vi "Universial XsYa.vi"() -> ()   [LabVIEW 2023]
uses:
  <vilib>/Utility/file.llb/Write Delimited Spreadsheet (DBL).vi
panel:
  in  "Status":enum32{"Measurement Status"}(tab)
  in  "Comments":string="See the below notes for this measurement.\n\nSR785 Status:Fre Span 51200.000000\n Hz; Center Fre 25600.000000\n Hz; Points(0 for 101, 1 for 201, 2 for 401 3 for 801): 2\n; Start, End Fre: 0.000000\n, 51200.000000\nHz; Unit y: dBVpk\n;\n"
  out "Current FIeld":dbl=0.5
  out "Current Current":dbl=2.5
  out "error out":errorcluster
  in  "Response Control":enum32{"cRIO slow V", "SR785"}(tab)=enum."SR785"
  in  "Channel":string(combo)="AI0"
  in  "Average":i32=1000
  out "FFT record time s":dbl=0.015625 caption="Delay Time (s)"
  in  "SR785 VISA":string="GPIB0::10::INSTR"
  in  "Display data":i32(ring) items=["Display A", "Display B"]
  in  "Center Hz":dbl=25000.0 format="%^.2e"
  in  "Span Hz":dbl=50000.0 format="%^.2e"
  in  "Resolution":i32(ring)=3 items=["100", "200", "400", "800"]
  out "CRIO pipe":T1={"DAQ_CMD_Writer endpoint"="DAQ_CMD_Writer", "DAQ_AI_Reader endpoint"="DAQ_AI_Reader", "vi reference"=refnum, "application reference"=refnum}
  in  "Excitation control":enum32{"B", "I"}(tab)
  in  "B Origin":dbl=-1.5 format="%#_13g"
  in  "B Radius":dbl=2.0 format="%#_13g"
  in  "B step":dbl=0.1 format="%#_13g"
  in  "B Ramp first":bool=TRUE
  in  "B Ramp type":string(combo)="Range"
  in  "Magnet Device Select":string(combo)="Elsa Magnet mT"
  in  "Field Rate mT per sec":dbl=0.1 format="%#_13g"
  in  "scale":dbl=1.0
  in  "I Origin":dbl format="%#_13g"
  in  "I step":dbl=0.05 format="%#_13g"
  in  "I Radius":dbl=2.5 format="%#_13g"
  in  "I Ramp first":bool=TRUE
  in  "I Ramp type":string(combo)="Range"
  in  "I Device Select":string(combo)="cRIO Slow"
  in  "AO Channel":string(combo)="AO0"
  in  "Book number":i32=684
  in  "parent data folder":path=path "C:/Users/gyue/Box/Guang Yue uiuc research box folder/data/Contour plot"
  # "This VI control measurements of multiple indenpent variable (Xs, such as B, I) and single channel data array (Yarray, FFT, V curve etc.)"
  # "Data structure: time-para.xml for all VI controls value, para.dat contains dimensions of data in form (x1 numbers, x2 numbers\\n y1 numbers, y2, numbers), field.dat contains lines of independent variables at each measurement, data.dat contains measurment data line, one measurement per line or group of lines."
  # "Attation: The actuall frequency may different from set value, check the Comments control."
  # "value in uA x scale=raw"
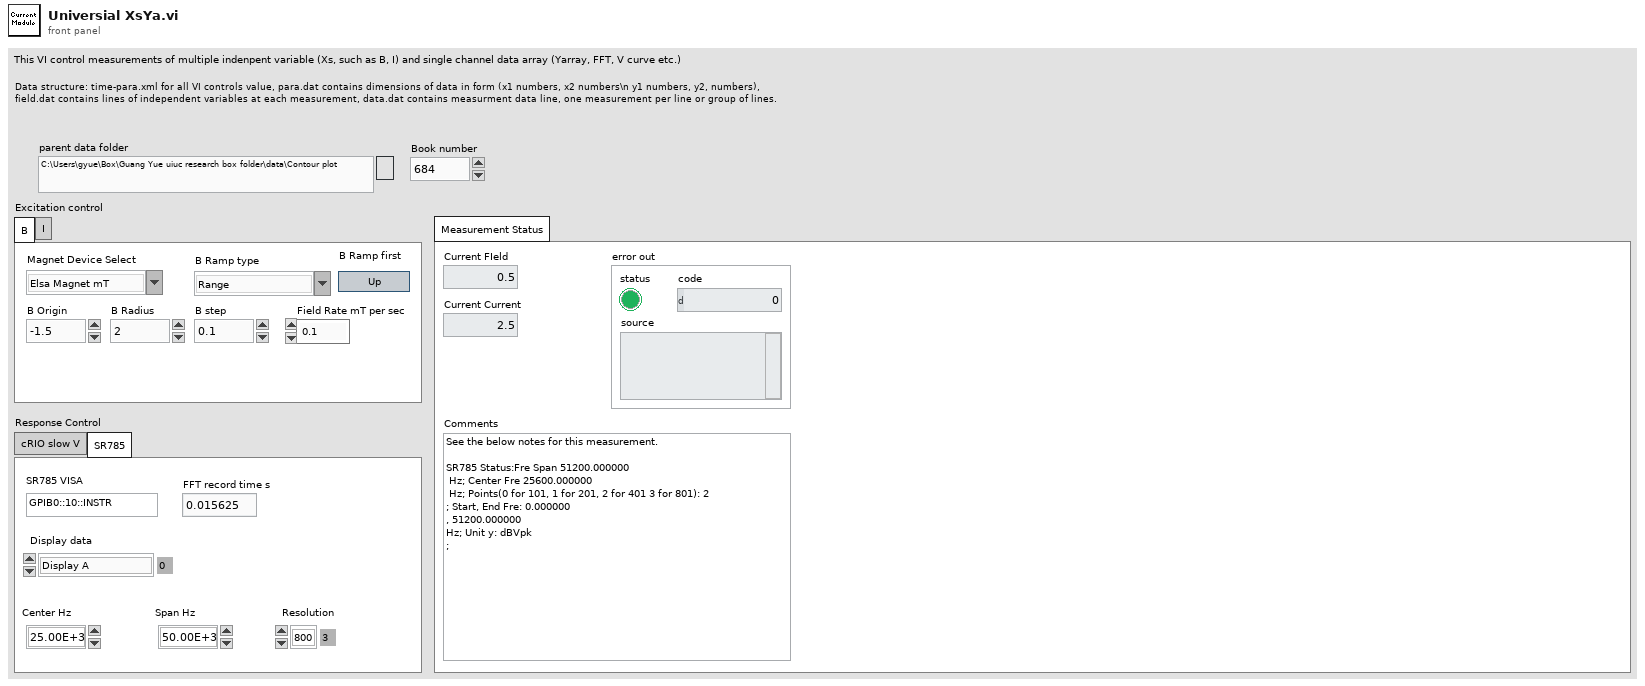
[diagram p1: front panel]
types:
  T1 = cluster{"DAQ_CMD_Writer endpoint":refnum<k21>, "DAQ_AI_Reader endpoint":refnum<k21>, "vi reference":refnum<vi>, "application reference":refnum<vi>}
  T2 = cluster{"AI0":dbl, "AI1":dbl, "AI2":dbl, "AI3":dbl}
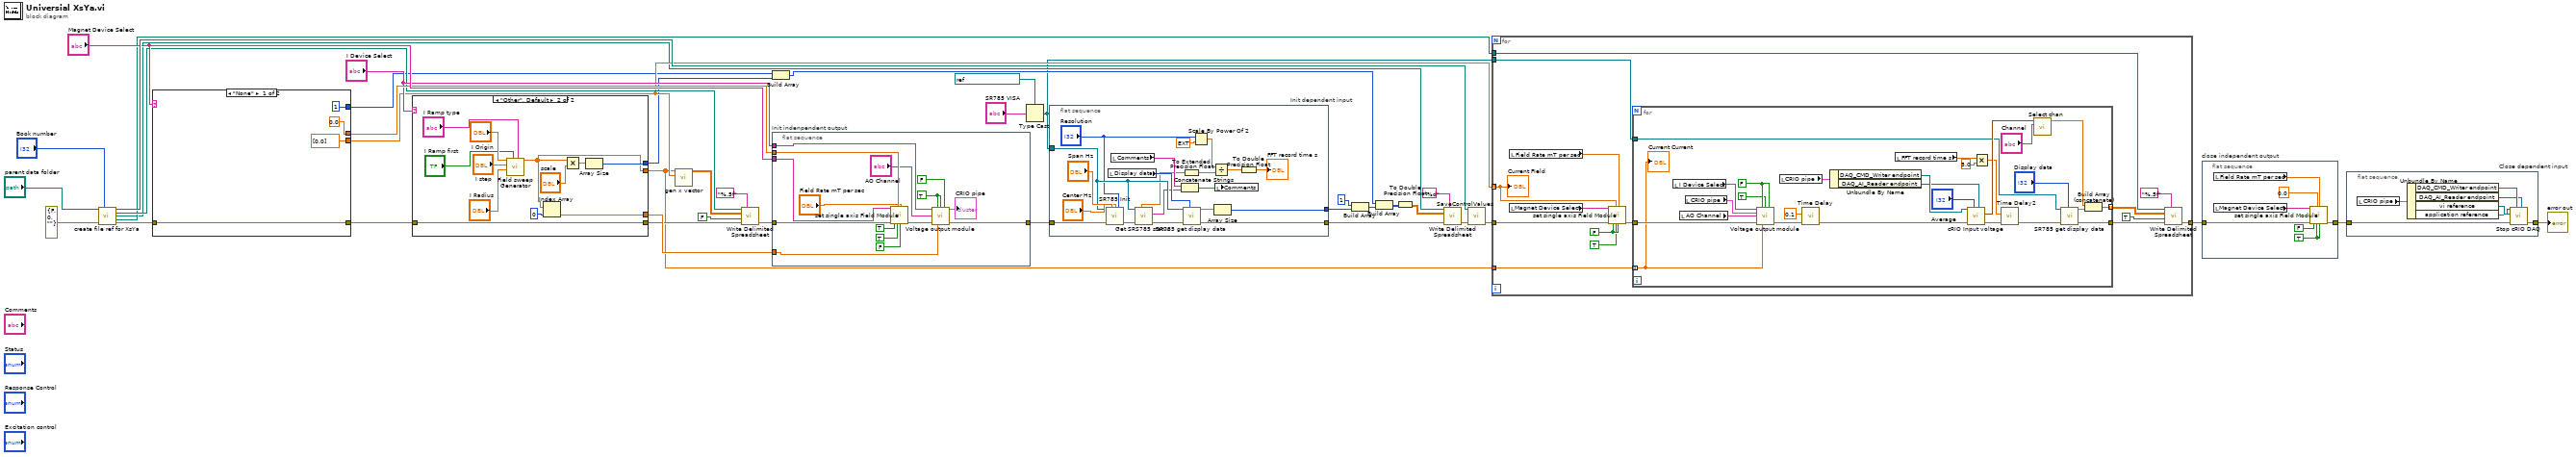
[diagram p0: block diagram]
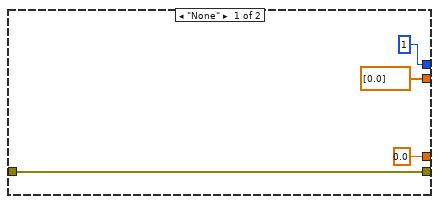
[diagram p2: hidden frame]
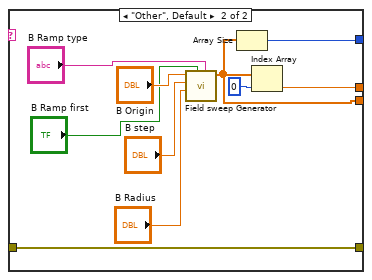
[diagram p3: hidden frame]
diagram:
  n1 = call "create file ref for XsYa.vi"("parent data folder"="parent data folder", "Book number"="Book number", "error in"=errorcluster {"status"=FALSE, "code"=0, "source"=""}) -> ("xml path"=w36:path, "field dat"=w27:path, "para dat"=w16:path, "data dat"=w21:path, "error out"=w3:errorcluster)  [unwired: 8 in]
  n2 = case shown="\"None\"" "Magnet Device Select" {
    tunnel: [0.0 w47] -> w34
    tunnel: w3 -> [w42 w46]
    tunnel: [w42 w46] -> w31
    tunnel: [dbl[] [0.0] ("output array") w45] -> w24
    tunnel: [1 w44] -> w14
    frame "None" {
    }
    frame "Other", Default {
      n3 = call "Field sweep Generator.vi"("Ramp type"="B Ramp type", "Ramp up first T"="B Ramp first", "Field Radius"="B Radius", "Field step"="B step", "Field Origin"="B Origin") -> ("output array"=w45:dbl[])  [unwired: 6 in]
      n4 = Array Size(array=w45) -> (size(s)=w44:i32)
      n5 = Index Array(array=w45, index=0) -> (element=w47:dbl)
    }
  }
  n6 = case shown="\"Other\", Default" "I Device Select" {
    tunnel: [0.0 w63] -> w32
    tunnel: w31 -> [w56 w62]
    tunnel: [w56 w62] -> w30
    tunnel: [dbl[] [0.0] ("output array") w58] -> w23
    tunnel: [1 w59] -> w13
    frame "None" {
    }
    frame "Other", Default {
      n7 = call "Field sweep Generator.vi"("Ramp type"="I Ramp type", "Ramp up first T"="I Ramp first", "Field Radius"="I Radius", "Field step"="I step", "Field Origin"="I Origin") -> ("output array"=w58:dbl[])  [unwired: 6 in]
      n8 = Index Array(array=w58, index=0) -> (element=w63:dbl)
      n9 = Multiply(x=w58, y="scale") -> (x*y=w60:dbl[])
      n10 = Array Size(array=w60) -> (size(s)=w59:i32)
    }
  }
  n11 = call "gen x vector.vi"("B"=w24, "I"=w23) -> ("Array"=w25:dbl[][])  [unwired: 9 in]
  n12 = call-poly <vilib>:"Write Delimited Spreadsheet.vi"("file path (dialog if empty)"=w27, "format (%.3f)"="%.5f", "2D data"=w25, "append to file? (new file:F)"=FALSE, "error in (no error)"=w30) -> ("error out"=w29:errorcluster)  [unwired: 9 in, 1 out]
  n13 = Build Array(w14, w13) -> (w12:i32[])
  n14 = flat-sequence "Init indenpendent output" {
    tunnel: w29 -> [w72]
    tunnel: w34 -> [w81]
    tunnel: "Magnet Device Select" -> [w80]
    tunnel: "I Device Select" -> [w79]
    tunnel: w32 -> [w78]
    tunnel: [w71] -> w22
    frame #0 {
      w77 = TRUE ("Init")
      n15 = call "set single axis Field Module.vi"("Field Device Select"=w80, "error in (no error)"=w72, "Init"=TRUE, "Field Target mT or dBm"=w81, "Exec"=TRUE, "Field Rate mT per sec"="Field Rate mT per sec", "final"=FALSE) -> ("error out"=w75:errorcluster)  [unwired: 12 in]
      n16 = call "Voltage output module.vi"("Device Select"=w79, "Init"=w77, "Exec"=w77, "finish up"=FALSE, "AO Channel"="AO Channel", "Error In"=w75, "Voltage"=w78) -> ("current Control pipe"=→"CRIO pipe":T1, "Error out"=w71:errorcluster)  [unwired: 7 in]
    }
  }
  n17 = Type Cast(type=refnum<visa-resource-name> "GPIB0::10::INSTR" ("SR785 VISA"), x="SR785 VISA") -> (*(type *) &x=w7:refnum<visa-resource-name>)
  n18 = flat-sequence "Init dependent input" {
    tunnel: w22 -> [w101]
    tunnel: [w85] -> w4
    tunnel: w7 -> [w98]
    tunnel: [w102] -> w6
    frame #0 {
      n19 = call "SR785 Init.vi"("VISA resource name"=w98, "Center (51.2E+3 Hz)"="Center Hz", "Span (102.4E+3 Hz)"="Span Hz", "Resolution (2: 400)"="Resolution", "error in (no error)"=w101) -> ("error out"=w87:errorcluster)  [unwired: 10 in]
      n20 = local read "Display data"() -> (w104:i32)
      n21 = local read "Comments"() -> (w97:string)
      n22 = call "Get SRS785 status.vi"("error in (no error)"=w87, "VISA resource name"=w98) -> ("error out"=w86:errorcluster, "concatenated string"=w96:string, "Frequency Span"=w91:dbl)  [unwired: 3 in, 4 out]
      n23 = Concatenate Strings(w97, w96) -> (w95:string)
      n24 = call "SR785 get display data.vi"("Display (0: Display A)"=w104, "error in (no error)"=w86, "VISA resource name"=w98) -> ("error out"=w85:errorcluster, "Waveform Graph"=w103:dbl[])  [unwired: 7 in]
      n25 = To Extended Precision Float(1:w91) -> (0:w90:ext)
      n26 = Scale By Power Of 2(n="Resolution", x=ext 100.0) -> (x*2^n=w92:ext)
      n27 = Divide(x=w92, y=w90) -> (x/y=w89:ext)
      n28 = Array Size(array=w103) -> (size(s)=w102:i32)
      n29 = local write "Comments"(w95) -> ()
      n30 = To Double Precision Float(number=w89) -> (double precision float=→"FFT record time s":dbl)
    }
  }
  n31 = Build Array(1 ("element"), w6) -> (w10:i32[])
  n32 = Build Array(w12, w10) -> (w9:i32[][])
  n33 = To Double Precision Float(number=w9) -> (double precision float=w8:dbl[][])
  n34 = call-poly <vilib>:"Write Delimited Spreadsheet.vi"("file path (dialog if empty)"=w16, "format (%.3f)"="%d", "2D data"=w8, "error in (no error)"=w4) -> ("error out"=w2:errorcluster)  [unwired: 10 in, 1 out]
  n35 = call "SaveControlValues.vi"("XML File Path"=w36, "error in (no error)"=w2) -> ("error out"=w1:errorcluster)  [unwired: 8 in]
  n36 = for {
    tunnel: w24 -> [w115] mode=indexing
    tunnel: w1 -> [w119]
    tunnel: w23 -> [w113]
    tunnel: w7 -> [w111]
    tunnel: w21 -> [w110]
    tunnel: [w105] -> w5
    w117 = FALSE ("Init")
    n37 = local read "Magnet Device Select"() -> (w118:string)
    n38 = local read "Field Rate mT per sec"() -> (w114:dbl)
    n39 = call "set single axis Field Module.vi"("Field Device Select"=w118, "error in (no error)"=w119, "Init"=w117, "Field Target mT or dBm"=w115, "Exec"=TRUE, "Field Rate mT per sec"=w114, "final"=w117) -> ("error out"=w112:errorcluster)  [unwired: 12 in]
    n40 = for {
      tunnel: w113 -> [w140] mode=indexing
      tunnel: w112 -> [w146]
      tunnel: w111 -> [w128]
      tunnel: [w125] -> w108 mode=indexing
      tunnel: [w124] -> w107
      w143 = FALSE ("Init")
      n41 = local read "I Device Select"() -> (w145:string)
      n42 = local read "AO Channel"() -> (w144:string)
      n43 = local read "CRIO pipe"() -> (w141:T1)
      n44 = call "Voltage output module.vi"("Device Select"=w145, "Init"=w143, "Exec"=TRUE, "finish up"=w143, "Input Control pipe"=w141, "AO Channel"=w144, "Error In"=w146, "Voltage"=w140) -> ("Error out"=w139:errorcluster)  [unwired: 6 in, 1 out]
      n45 = local read "CRIO pipe"() -> (w136:T1)
      n46 = call "Time Delay"("error in (no error)"=w139, "Delay Time (s)"=0.1) -> ("error out"=w138:errorcluster)  [unwired: 9 in]
      n47 = Unbundle By Name(w136) -> ("DAQ_CMD_Writer endpoint"=w135:refnum<k21>, "DAQ_AI_Reader endpoint"=w134:refnum<k21>)
      n48 = local read "FFT record time s"() -> (w122:dbl)
      n49 = call "cRIO Input voltage.vi"("DAQ_AI_Reader endpoint"=w134, "Average"="Average", "error in (no error)"=w138, "DAQ_CMD_Writer endpoint"=w135) -> ("error out"=w132:errorcluster, "output cluster"=w131:T2)  [unwired: 5 in, 1 out]
      n50 = Multiply(x=w122, y=5.0) -> (x*y=w121:dbl)
      n51 = call "Time Delay2"("error in (no error)"=w132, "Delay Time (s)"=w121) -> ("error out"=w129:errorcluster)  [unwired: 9 in]
      n52 = call "Select chan.vi"("Channel"="Channel", "output cluster"=w131) -> ("Output"=w126:dbl)  [unwired: 9 in]
      n53 = call "SR785 get display data.vi"("Display (0: Display A)"="Display data", "error in (no error)"=w129, "VISA resource name"=w128) -> ("error out"=w124:errorcluster, "Waveform Graph"=w123:dbl[])  [unwired: 7 in]
      n54 = Build Array (concatenate)(w126, w123) -> (w125:dbl[])
      "Current Current" <- w140
    }
    n55 = call-poly <vilib>:"Write Delimited Spreadsheet.vi"("file path (dialog if empty)"=w110, "format (%.3f)"="%.5f", "2D data"=w108, "append to file? (new file:F)"=TRUE, "error in (no error)"=w107) -> ("error out"=w105:errorcluster)  [unwired: 9 in, 1 out]
    "Current FIeld" <- w115
  }
  n56 = flat-sequence "close independent output" {
    tunnel: w5 -> [w153]
    tunnel: [w152] -> w18
    frame #0 {
      w150 = TRUE ("Exec")
      n57 = local read "Magnet Device Select"() -> (w149:string)
      n58 = local read "Field Rate mT per sec"() -> (w147:dbl)
      n59 = call "set single axis Field Module.vi"("Field Device Select"=w149, "error in (no error)"=w153, "Init"=FALSE, "Field Target mT or dBm"=0.0 ("Field Target mT"), "Exec"=w150, "Field Rate mT per sec"=w147, "final"=w150) -> ("error out"=w152:errorcluster)  [unwired: 12 in]
    }
  }
  n60 = flat-sequence "Close dependent input" {
    tunnel: w18 -> [w160]
    tunnel: [w159] -> w17
    frame #0 {
      n61 = local read "CRIO pipe"() -> (w158:T1)
      n62 = Unbundle By Name(w158) -> ("DAQ_CMD_Writer endpoint"=w157:refnum<k21>, "DAQ_AI_Reader endpoint"=w156:refnum<k21>, "vi reference"=w155:refnum<vi>, "application reference"=w154:refnum<vi>)
      n63 = call "Stop cRIO DAQ.vi"("DAQ_AI_Reader endpoint"=w156, "DAQ_CMD_Writer endpoint"=w157, "error in (no error)"=w160, "VI reference"=w155, "application reference"=w154) -> ("error out"=w159:errorcluster)  [unwired: 6 in]
    }
  }
  "error out" <- w17
